vi "GetInterfacesOfClass.vi"(8 "error in":errorcluster, 11 "LvClassRefIn":refnum<vi>) -> (0 "error out":errorcluster, 1 "Interfaces(MethodsImplemented)":cluster{"Methods":string[]}[](array[cluster]), 2 "Interfaces(path)":path[](array[path]), 3 "LvClassRefOut":refnum<vi>)   [LabVIEW 2020, in "InterfaceLibrary.lvlib"]
uses:
  <resource>/Framework/Providers/Open_GDS/ClassProviders/Common/InterfaceLibrary/InterfaceLibrary.lvlib
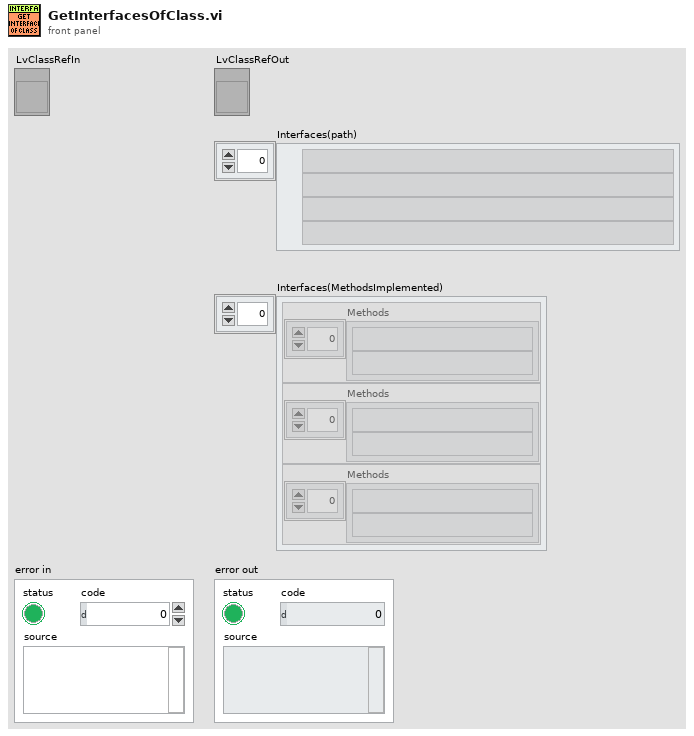
[diagram p1: front panel]
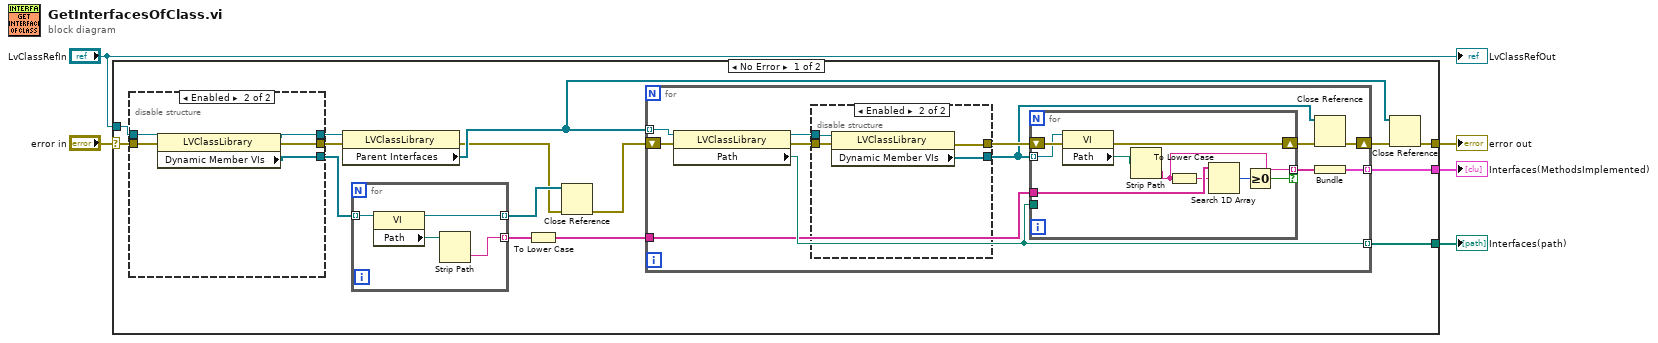
[diagram p0: block diagram]
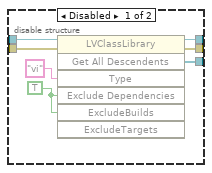
[diagram p2: hidden frame]
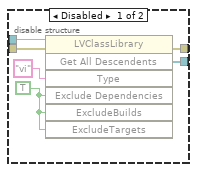
[diagram p3: hidden frame]
diagram:
  n1 = case shown="No Error" "error in" {
    selector: "error in" -> [w16 w68]
    tunnel: "LvClassRefIn" -> [w15 _]
    tunnel: [w10 w68] -> w4
    tunnel: [w19 _] -> w1
    tunnel: [w18 _] -> w2
    frame No Error {
      n2 = disable-structure shown="Enabled" {
        disable-tunnel: w16 -> [w25 w31]
        disable-tunnel: w15 -> [w24 w32]
        disable-tunnel: [w23 w29] -> w14
        disable-tunnel: [w22 w28] -> w13
        disable-tunnel: [w21 w30] -> w6
        frame Disabled {
          w26 = TRUE ("ExcludeDependencies")
          n3 = invoke class="LVClassLibrary" method="Get All Descendents"(reference=w24, error in=w25, "Type"="vi", "Exclude Dependencies"=w26, "ExcludeBuilds"=w26) -> (reference out=w21:refnum<vi>, error out=w23:errorcluster, "All Descendents"=w22:refnum<vi>[])  [unwired: 2 in, 4 out]
        }
        frame Enabled {
          n4 = property class="LVClassLibrary"(reference=w32, error in=w31) -> (reference out=w30:refnum<vi>, error out=w29:errorcluster, "Dynamic Member VIs"=w28:refnum<vi>[])
        }
      }
      n5 = property class="LVClassLibrary"(reference=w6, error in=w14) -> (error out=w8:errorcluster, "Parent Interfaces"=w17:refnum<vi>[])  [unwired: 1 out]
      n6 = for {
        tunnel: w13 -> [w36] mode=indexing
        tunnel: [w33] -> w12 mode=indexing
        tunnel: [w35] -> w9 mode=indexing
        n7 = property class="VI"(reference=w36) -> (reference out=w35:refnum<vi>, "Path"=w34:path)  [unwired: 1 in, 1 out]
        n8 = Strip Path(path=w34) -> (name=w33:string)  [unwired: 1 out]
      }
      n9 = To Lower Case(string=w12) -> (all lower case string=w11:string[])
      n10 = Close Reference(reference=w9, error in (no error)=w8) -> (error out=w7:errorcluster)
      n11 = for {
        tunnel: w17 -> [w41] mode=indexing
        shift-right: [w37] -> w20
        shift-left: w7 -> [w48]
        tunnel: [w42] -> w19 mode=indexing
        tunnel: [w38] -> w18 mode=indexing
        tunnel: w11 -> [w40]
        n12 = property class="LVClassLibrary"(reference=w41, error in=w48) -> (reference out=w46:refnum<vi>, error out=w47:errorcluster, "Path"=w42:path)
        n13 = disable-structure shown="Enabled" {
          disable-tunnel: w47 -> [w54 w57]
          disable-tunnel: w46 -> [w53 w58]
          disable-tunnel: [w50 w56] -> w45
          disable-tunnel: [w49 w55] -> w43
          frame Disabled {
            w52 = TRUE ("ExcludeDependencies")
            n14 = invoke class="LVClassLibrary" method="Get All Descendents"(reference=w53, error in=w54, "Type"="vi", "Exclude Dependencies"=w52, "ExcludeBuilds"=w52, "ExcludeTargets"=w52) -> (error out=w50:errorcluster, "All Descendents"=w49:refnum<vi>[])  [unwired: 1 in, 5 out]
          }
          frame Enabled {
            n15 = property class="LVClassLibrary"(reference=w58, error in=w57) -> (error out=w56:errorcluster, "Dynamic Member VIs"=w55:refnum<vi>[])  [unwired: 1 out]
          }
        }
        n16 = for {
          tunnel: w43 -> [w66] mode=indexing
          shift-right: [w65] -> w44
          shift-left: w45 -> [w67]
          tunnel: w42 -> [_]
          tunnel: w40 -> [w64]
          tunnel: [w59] -> w39 mode=indexing if=w61
          n17 = property class="VI"(reference=w66, error in=w67) -> (error out=w65:errorcluster, "Path"=w60:path)  [unwired: 1 out]
          n18 = Strip Path(path=w60) -> (name=w59:string)  [unwired: 1 out]
          n19 = To Lower Case(string=w59) -> (all lower case string=w63:string)
          n20 = Search 1D Array(1D array=w64, element=w63) -> (index of element=w62:i32)  [unwired: 1 in]
          n21 = Greater Or Equal To 0?(x=w62) -> (x >= 0?=w61:bool)
        }
        n22 = Close Reference(reference=w43, error in (no error)=w44) -> (error out=w37:errorcluster)
        n23 = Bundle(w39) -> (w38:cluster{string[]})  [unwired: 1 in]
      }
      n24 = Close Reference(reference=w17, error in (no error)=w20) -> (error out=w10:errorcluster)
    }
    frame Error {
    }
  }
  "error out" <- w4
  "Interfaces(path)" <- w1
  "Interfaces(MethodsImplemented)" <- w2
  "LvClassRefOut" <- "LvClassRefIn"
